vi "Read Views.vi"(8 "error in (no error)":errorcluster, 11 "GUI Container Actor in":refnum<class "GUI Container Actor.lvclass">) -> (0 "error out":errorcluster, 3 "GUI Container Actor out":refnum<class "GUI Container Actor.lvclass">)   [LabVIEW 2017, in "GUI Views.lvlib" / "GUI Container Actor.lvclass"]
uses:
  GUI Container Actor.lvclass
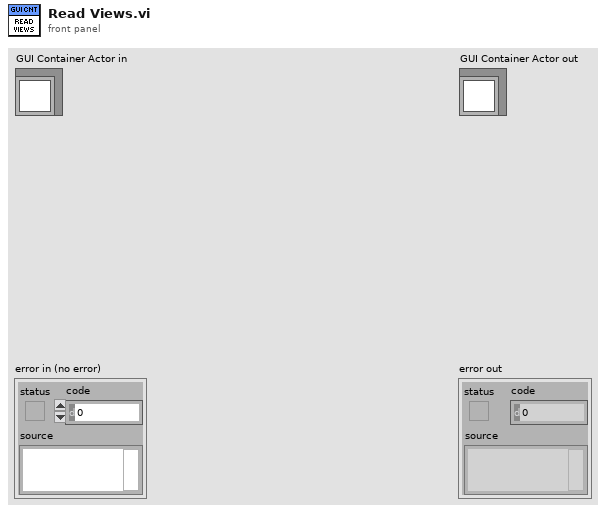
[diagram p1: front panel]
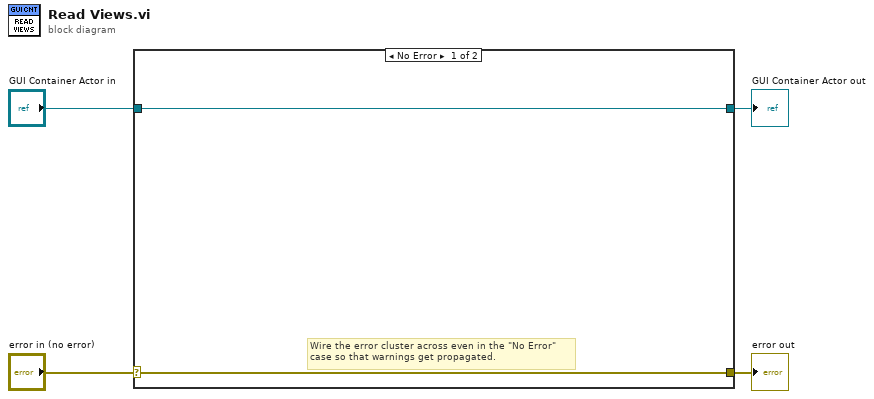
[diagram p0: block diagram]
diagram:
  n1 = case shown="No Error" "error in (no error)" {
    selector: "error in (no error)" -> [w5 w8]
    tunnel: [w5 w8] -> w3
    tunnel: [w6 w7] -> w1
    tunnel: "GUI Container Actor in" -> [w6 w7]
    frame No Error {
      # "Wire the error cluster across even in the \"No Error\"\ncase so that warnings get propagated."
    }
    frame Error {
    }
  }
  "error out" <- w3
  "GUI Container Actor out" <- w1
